vi "Clear.vi"(8 "error in (no error)":errorcluster, 11 "Mock Voltage Output In":refnum<class "Mock Voltage Output.lvclass">) -> (0 "error out":errorcluster, 3 "Mock Voltage Output Out":refnum<class "Mock Voltage Output.lvclass">)   [LabVIEW 2020, in "High Level PSU With Tests.lvlib" / "Mock Voltage Output.lvclass"]
uses:
  Mock Voltage Output.lvclass
  Mock Voltage Output.lvclass/Mock Voltage Output.ctl
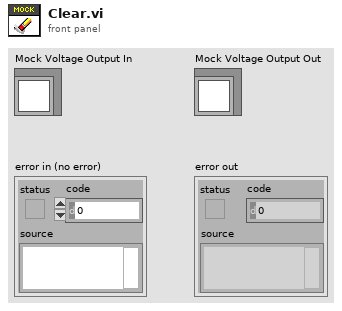
[diagram p1: front panel]
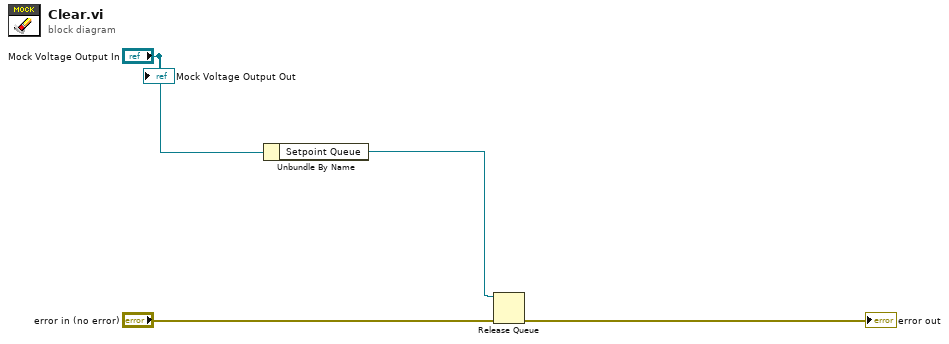
[diagram p0: block diagram]
diagram:
  n1 = Unbundle By Name("Mock Voltage Output In") -> ("Setpoint Queue"=w1:refnum<queue>)
  n2 = Release Queue(queue=w1, error in (no error)="error in (no error)") -> (error out=→"error out":errorcluster)  [unwired: 1 in, 2 out]
  "Mock Voltage Output Out" <- "Mock Voltage Output In"
